vi "Enc_mm (SubVI).vi"(11 "EncodersParam1":u64) -> (3 "Numeric":ext)   [LabVIEW 2017]
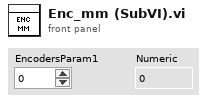
[diagram p1: front panel]
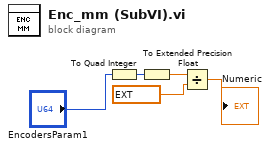
[diagram p0: block diagram]
diagram:
  n1 = To Quad Integer(1:"EncodersParam1") -> (0:w5:i64)
  n2 = To Extended Precision Float(1:w5) -> (0:w2:ext)
  n3 = Divide(x=w2, y=ext 1000000.0) -> (x/y=→"Numeric":ext)
